vi "4 Bit BDD.vi"() -> ()   [LabVIEW 2012]
panel:
  out "9":bool
  out "8":bool
  out "7":bool
  out "6":bool
  out "5":bool
  out "4":bool
  out "3":bool
  in  "d":bool
  out "2":bool
  out "1":bool
  out "0":bool
  in  "c":bool
  in  "b":bool
  in  "a":bool
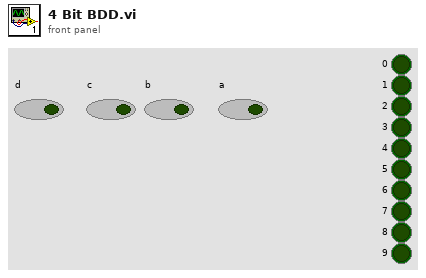
[diagram p1: front panel]
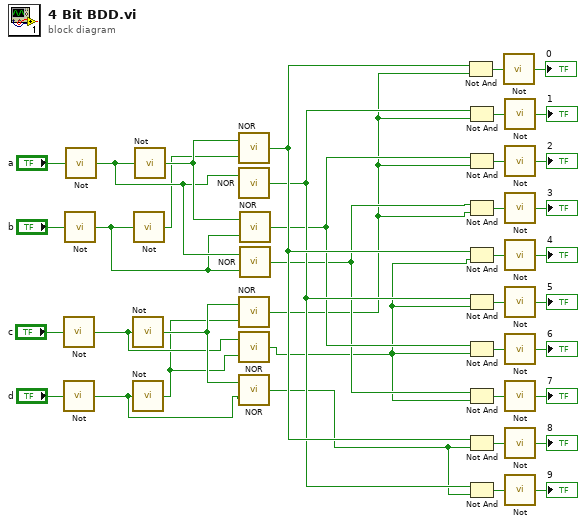
[diagram p0: block diagram]
diagram:
  n1 = call "Not.vi"("In"="c") -> ("Out"=w30:bool)
  n2 = call "Not.vi"("In"="d") -> ("Out"=w29:bool)
  n3 = call "Not.vi"("In"="b") -> ("Out"=w32:bool)
  n4 = call "Not.vi"("In"="a") -> ("Out"=w34:bool)
  n5 = call "Not.vi"("In"=w30) -> ("Out"=w31:bool)
  n6 = call "Not.vi"("In"=w29) -> ("Out"=w1:bool)
  n7 = call "Not.vi"("In"=w32) -> ("Out"=w33:bool)
  n8 = call "Not.vi"("In"=w34) -> ("Out"=w35:bool)
  n9 = call "NOR.vi"("b"=w33, "a"=w35) -> ("x"=w8:bool)
  n10 = call "NOR.vi"("a"=w34) -> ("x"=w7:bool)  [unwired: 1 in]
  n11 = call "NOR.vi"("b"=w1, "a"=w31) -> ("x"=w4:bool)
  n12 = call "NOR.vi"("b"=w1, "a"=w30) -> ("x"=w3:bool)
  n13 = call "NOR.vi"("b"=w29, "a"=w31) -> ("x"=w2:bool)
  n14 = call "NOR.vi"("b"=w32, "a"=w35) -> ("x"=w6:bool)
  n15 = call "NOR.vi"("b"=w32, "a"=w34) -> ("x"=w5:bool)
  n16 = Not And(1:w4, 2:w8) -> (0:w28:bool)
  n17 = Not And(1:w4, 2:w7) -> (0:w27:bool)
  n18 = Not And(1:w4, 2:w6) -> (0:w26:bool)
  n19 = Not And(1:w4, 2:w5) -> (0:w25:bool)
  n20 = Not And(1:w3, 2:w8) -> (0:w24:bool)
  n21 = Not And(1:w3, 2:w7) -> (0:w19:bool)
  n22 = Not And(1:w3, 2:w6) -> (0:w20:bool)
  n23 = Not And(1:w3, 2:w5) -> (0:w21:bool)
  n24 = Not And(1:w2, 2:w8) -> (0:w22:bool)
  n25 = Not And(1:w2, 2:w7) -> (0:w23:bool)
  n26 = call "Not.vi"("In"=w28) -> ("Out"=→"0":bool)
  n27 = call "Not.vi"("In"=w27) -> ("Out"=→"1":bool)
  n28 = call "Not.vi"("In"=w26) -> ("Out"=→"2":bool)
  n29 = call "Not.vi"("In"=w25) -> ("Out"=→"3":bool)
  n30 = call "Not.vi"("In"=w24) -> ("Out"=→"4":bool)
  n31 = call "Not.vi"("In"=w19) -> ("Out"=→"5":bool)
  n32 = call "Not.vi"("In"=w20) -> ("Out"=→"6":bool)
  n33 = call "Not.vi"("In"=w21) -> ("Out"=→"7":bool)
  n34 = call "Not.vi"("In"=w22) -> ("Out"=→"8":bool)
  n35 = call "Not.vi"("In"=w23) -> ("Out"=→"9":bool)
